vi "RxCalTest.vi"() -> ()   [LabVIEW 2015]
panel:
  in  "RxCalConfig":T1={"ExternalAtt"=0.0, "FreqHz"=5500000000.0, "Pwr"=0.0, "PacketNumber"=10000, "VISAName"="TCPIP0::10.144.41.48::inst0::INSTR", "WaveformName"="HT20MCS0.tdms", "Port"=5}
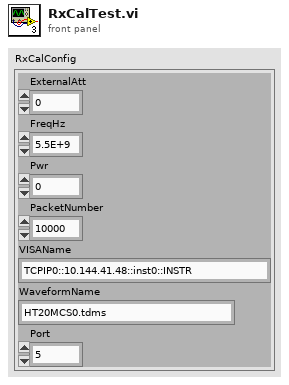
[diagram p1: front panel]
types:
  T1 = cluster{"ExternalAtt":dbl, "FreqHz":dbl, "Pwr":dbl, "PacketNumber":i32, "VISAName":string, "WaveformName":string, "Port":u32}
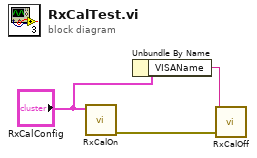
[diagram p0: block diagram]
diagram:
  n1 = call "RxCalOn.vi"("RxCalConfig"="RxCalConfig") -> ("error out"=w3:errorcluster)  [unwired: 10 in]
  n2 = Unbundle By Name("RxCalConfig") -> ("VISAName"=w1:string)
  n3 = call "RxCalOff.vi"("error in (no error)"=w3, "VISA"=w1) -> ()  [unwired: 9 in, 1 out]
